vi "12_1.vi"() -> ()   [LabVIEW 2018]
panel:
  out "Array 2":dbl[](array[numeric])
  out "Array":cluster{"North":dbl, "East":dbl}[](array[cluster])
  out "Manhattan Distance":dbl
  out "End Position":cluster{"North":dbl, "East":dbl}
  in  "Input":string
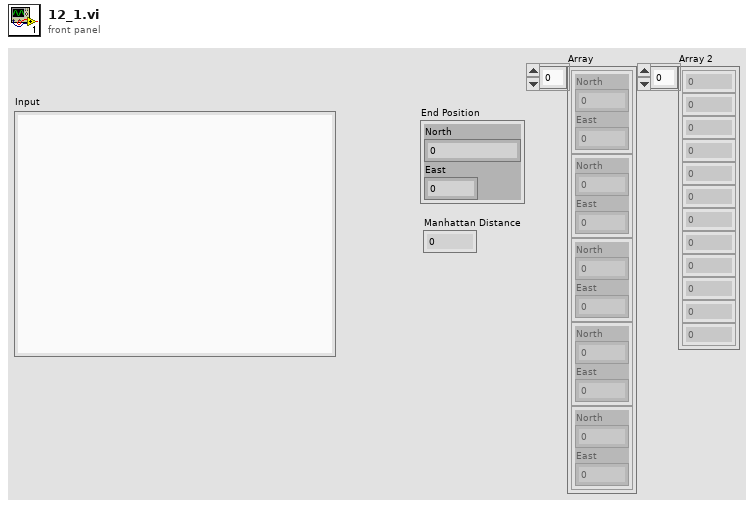
[diagram p1: front panel]
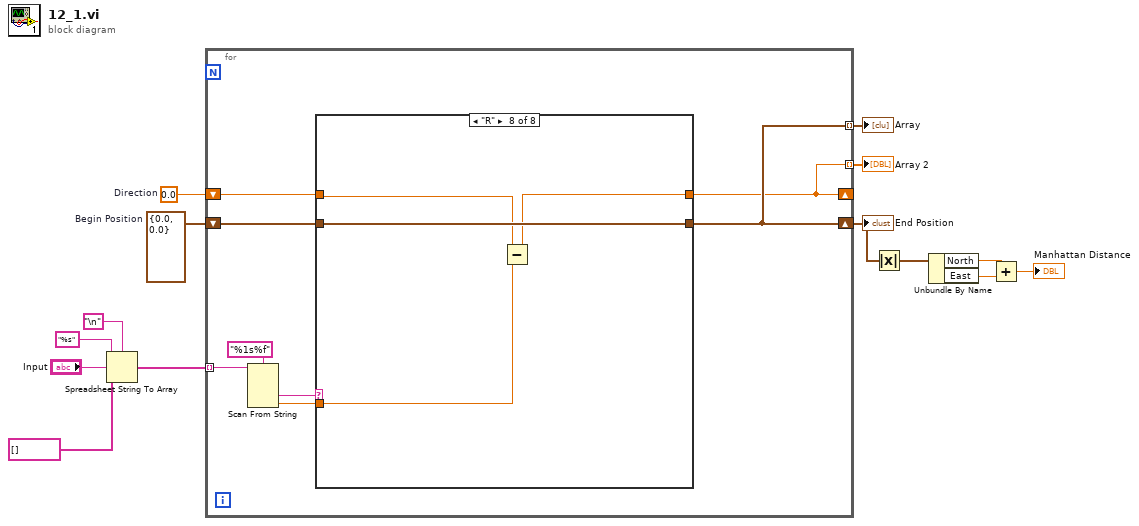
[diagram p0: block diagram]
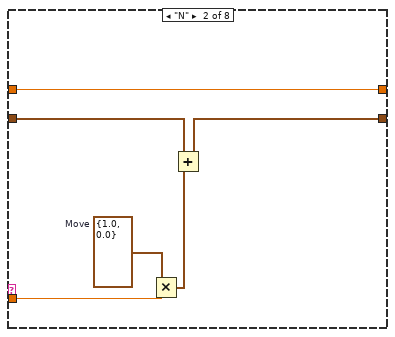
[diagram p3: hidden frame]
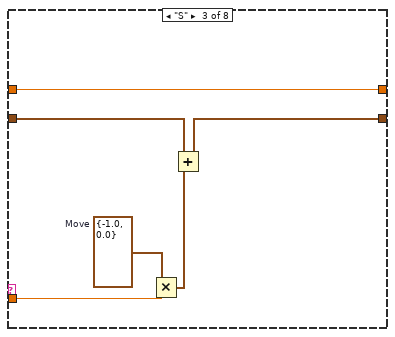
[diagram p4: hidden frame]
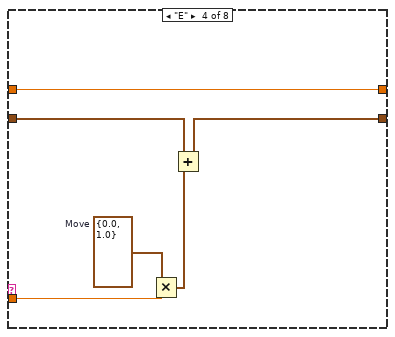
[diagram p5: hidden frame]
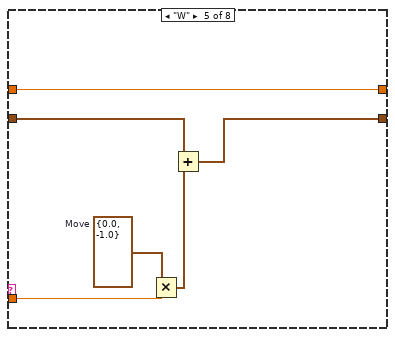
[diagram p6: hidden frame]
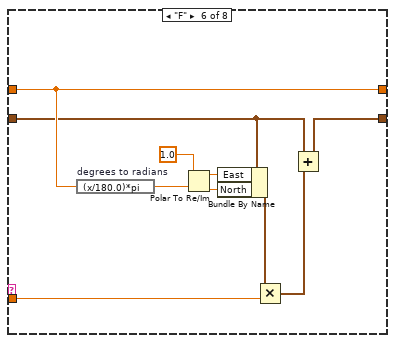
[diagram p7: hidden frame]
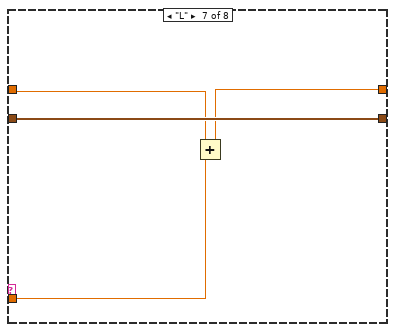
[diagram p8: hidden frame]
diagram:
  w3 = 0.0  # Direction
  w9 = cluster{"North":dbl, "East":dbl} {"North"=0.0, "East"=0.0}  # Begin Position
  n1 = Spreadsheet String To Array(delimiter (Tab)="\n", format string="%s", spreadsheet string="Input", array type (2D Dbl)=string[] []) -> (array=w10:string[])
  n2 = for {
    tunnel: w10 -> [w22] mode=indexing
    shift-right: [w15] -> _
    shift-left: w3 -> [w19]
    shift-right: [w16] -> w8
    shift-left: w9 -> [w18]
    tunnel: [w16] -> w2 mode=indexing
    tunnel: [w15] -> w1 mode=indexing
    n3 = Scan From String(format string="%1s%f", input string=w22) -> (output 1=w20:string, output 2=w17:dbl)  [unwired: 4 in, 3 out]
    n4 = case shown="\"R\"" w20 {
      tunnel: w19 -> [w24 w27 w33 w37 w43 w55 w61 w65]
      tunnel: w18 -> [w23 w25 w31 w38 w44 w51 w62 w66]
      tunnel: [w24 w27 w33 w37 w43 w55 w59 w63] -> w15
      tunnel: [w23 w26 w32 w39 w45 w56 w62 w66] -> w16
      tunnel: w17 -> [_ w30 w36 w42 w48 w58 w60 w64]
      frame Default {
      }
      frame "N" {
        w29 = cluster{"North":dbl, "East":dbl} {"North"=1.0, "East"=0.0}  # Move
        n5 = Multiply(x=w29, y=w30) -> (x*y=w28:cluster{"North":dbl, "East":dbl})
        n6 = Add(x=w25, y=w28) -> (x+y=w26:cluster{"North":dbl, "East":dbl})
      }
      frame "S" {
        w35 = cluster{"North":dbl, "East":dbl} {"North"=-1.0, "East"=0.0}  # Move
        n7 = Multiply(x=w35, y=w36) -> (x*y=w34:cluster{"North":dbl, "East":dbl})
        n8 = Add(x=w31, y=w34) -> (x+y=w32:cluster{"North":dbl, "East":dbl})
      }
      frame "E" {
        w41 = cluster{"North":dbl, "East":dbl} {"North"=0.0, "East"=1.0}  # Move
        n9 = Multiply(x=w41, y=w42) -> (x*y=w40:cluster{"North":dbl, "East":dbl})
        n10 = Add(x=w38, y=w40) -> (x+y=w39:cluster{"North":dbl, "East":dbl})
      }
      frame "W" {
        w47 = cluster{"North":dbl, "East":dbl} {"North"=0.0, "East"=-1.0}  # Move
        n11 = Multiply(x=w47, y=w48) -> (x*y=w46:cluster{"North":dbl, "East":dbl})
        n12 = Add(x=w44, y=w46) -> (x+y=w45:cluster{"North":dbl, "East":dbl})
      }
      frame "F" {
        n13 = expression code="(x/180.0)*pi" "degrees to radians"(w55) -> (w54:dbl)
        n14 = Polar To Re/Im(2:w54, 3:1.0) -> (0:w50:dbl, 1:w52:dbl)
        n15 = Bundle By Name(cluster=w51, "East"=w52, "North"=w50) -> (w49:cluster{"North":dbl, "East":dbl})
        n16 = Multiply(x=w49, y=w58) -> (x*y=w57:cluster{"North":dbl, "East":dbl})
        n17 = Add(x=w51, y=w57) -> (x+y=w56:cluster{"North":dbl, "East":dbl})
      }
      frame "L" {
        n18 = Add(x=w61, y=w60) -> (x+y=w59:dbl)
      }
      frame "R" {
        n19 = Subtract(x=w65, y=w64) -> (x-y=w63:dbl)
      }
    }
  }
  "End Position" <- w8
  "Array" <- w2
  "Array 2" <- w1
  n20 = Absolute Value(x=w8) -> (abs(x)=w7:cluster{"North":dbl, "East":dbl})
  n21 = Unbundle By Name(w7) -> ("North"=w5:dbl, "East"=w6:dbl)
  n22 = Add(x=w5, y=w6) -> (x+y=→"Manhattan Distance":dbl)
